vi "test-trapezoid-profile-timing-before-negative-goal.vi"() -> ()   [LabVIEW 2019]
uses:
  <vilib>/Rock Robotics/WPI/ThirdParty/JAS_Junk/TrajLib/TRAPEZOID_PROFILE_STATE.ctl
  <vilib>/Rock Robotics/WPI/ThirdParty/JAS_Junk/TrajLib/TRAPEZOID_PROFILE.ctl
  <vilib>/Rock Robotics/WPI/ThirdParty/JAS_Junk/TrajLib/TRAPEZOID_PROFILE_CONSTRAINT.ctl
  <vilib>/Rock Robotics/WPI/ThirdParty/JAS_Junk/TrajLib/TrapProfile_Direct.vi
  <vilib>/Rock Robotics/WPI/ThirdParty/JAS_Junk/TrajLib/TrapProfile_ShouldFlipAcceleration.vi
  <vilib>/Rock Robotics/WPI/ThirdParty/JAS_Junk/TrajLib/Trajectory_Library.lvlib
panel:
  out "ActualTime":dbl=-1.0
  out "PredictedTImeLeft":dbl
  out "TimeLeftGoal":dbl
  out "TimeLeftPos":dbl
  out "ReachedGoal":bool
  out "TotalTime":dbl
  out "TRAPEZOID_PROFILE":T1 {"Goal"."Velocity" format="%16_6e"; "Goal"."Position" format="%16_6e"; "Initial"."Velocity" format="%16_6e"; "Initial"."Position" format="%16_6e"; "Constraints"."MaxAcceleration" format="%16_6e"; "Constraints"."MaxVelocity" format="%16_6e"; "EndDecel" format="%16_6e"; "EndFullSpeed" format="%16_6e"; "EndAccel" format="%16_6e"}
  out "State":T3 {"Velocity" format="%16_6e"; "Position" format="%16_6e"}
  out "Waveform Chart":T4(graph)
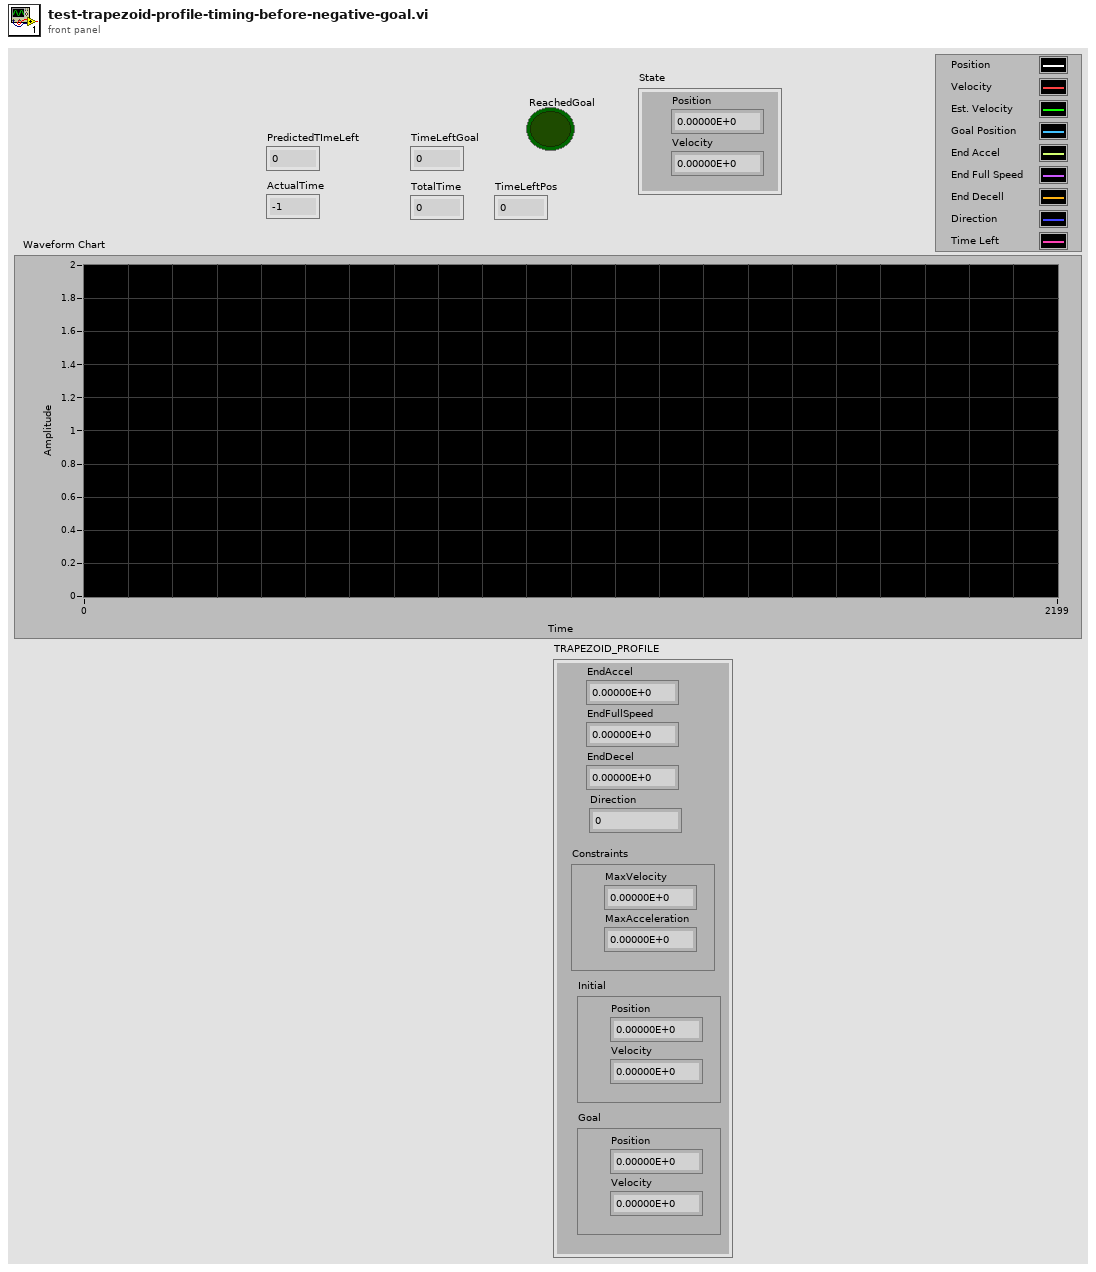
[diagram p1: front panel]
types:
  T1 = typedef "Trajectory_Library.lvlib/TRAPEZOID_PROFILE.ctl" = cluster{"EndAccel":dbl, "EndFullSpeed":dbl, "EndDecel":dbl, "Direction":i32, "Constraints":T2, "Initial":T3, "Goal":T3}
  T2 = typedef "Trajectory_Library.lvlib/TRAPEZOID_PROFILE_CONSTRAINT.ctl" = cluster{"MaxVelocity":dbl, "MaxAcceleration":dbl}
  T3 = typedef "Trajectory_Library.lvlib/TRAPEZOID_PROFILE_STATE.ctl" = cluster{"Position":dbl, "Velocity":dbl}
  T4 = cluster{"Position":dbl, "Velocity":dbl, dbl, "Position":dbl, "EndAccel":dbl, "EndFullSpeed":dbl, "EndDecel":dbl, "Direction":i32, "Position":dbl}
  T5 = cluster{"Position":dbl, "Velocity":dbl, dbl, "Position":dbl, "EndAccel":dbl, "EndFullSpeed":dbl, "EndDecel":dbl, "Direction":i32, "TimeLeft":dbl}
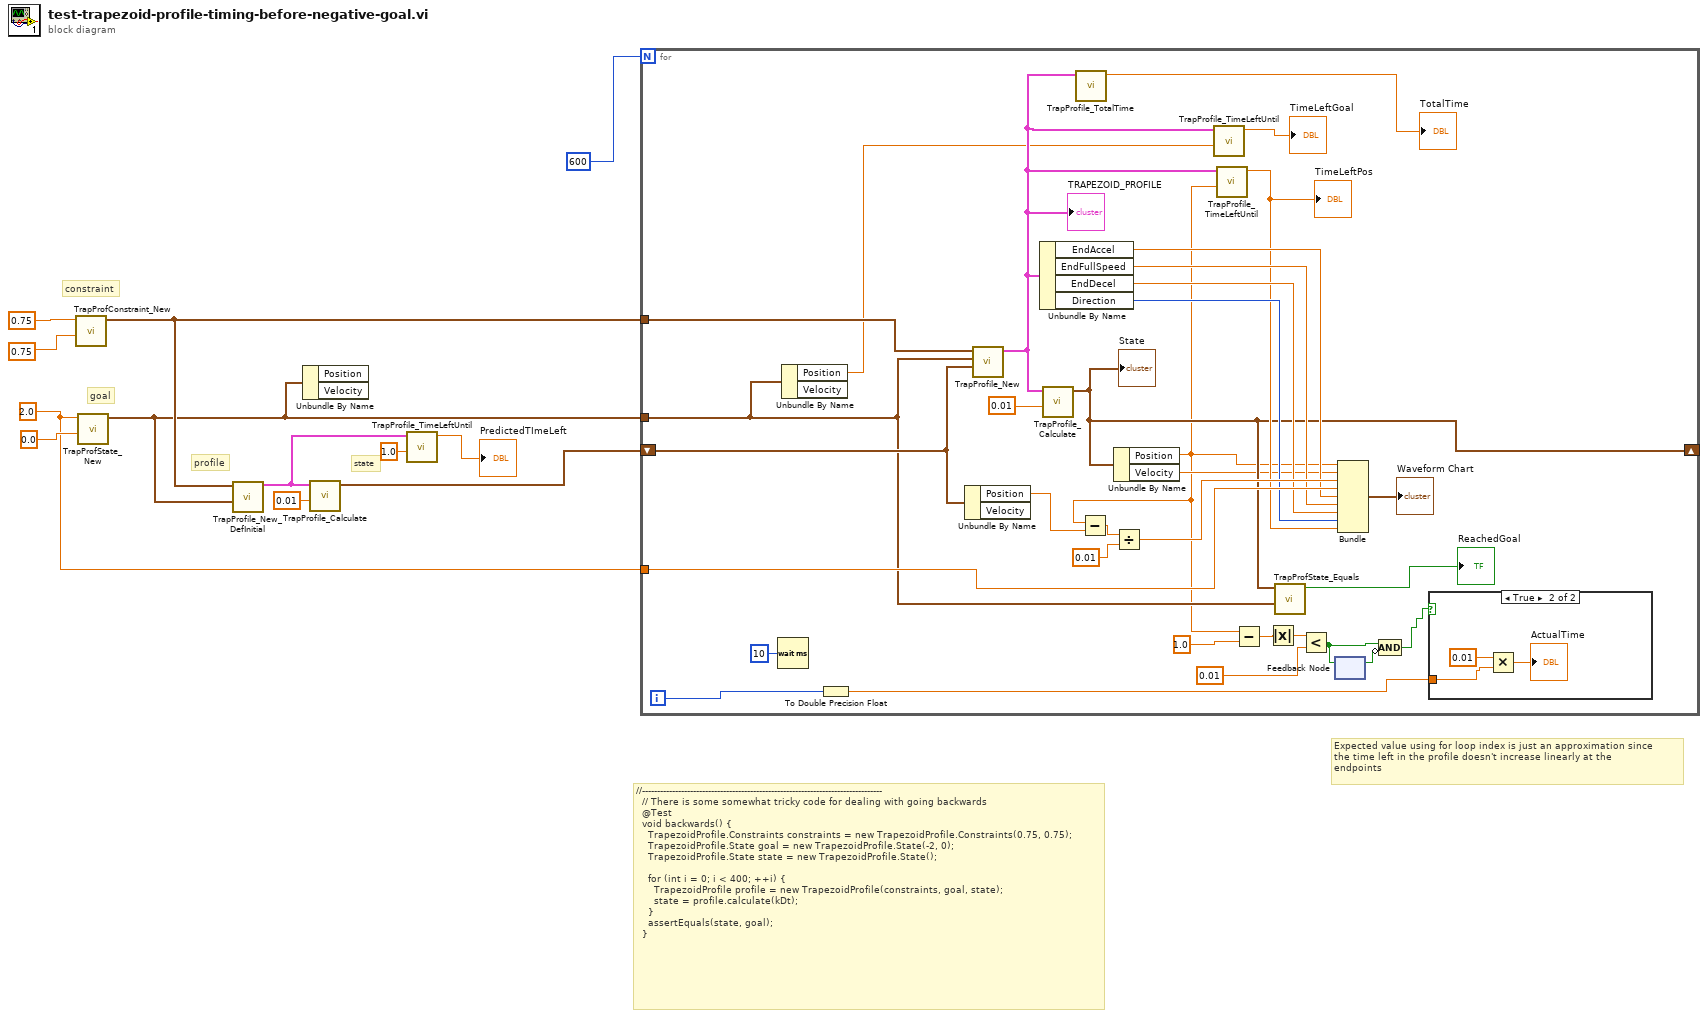
[diagram p0: block diagram]
diagram:
  w8 = 2.0 ("Position")
  # "Expected value using for loop index is just an approximation since\nthe time left in the profile doesn't increase linearly at the\nendpoints"
  # "profile"
  # "state"
  # "//--------------------------------------------------------------------------------\n  // There is some somewhat tricky code for dealing with going backwards\n  @Test\n  void backwards() {\n    TrapezoidProfile.Constraints constraints = new TrapezoidProfile.Constraints(0.75, 0.75);\n    TrapezoidProfile.State goal = new TrapezoidProfile.State(-2, 0);\n    TrapezoidProfile.State state = new TrapezoidProfile.State();\n\n    for (int i = 0; i < 400; ++i) {\n      TrapezoidProfile profile = new TrapezoidProfile(constraints, goal, state);\n      state = profile.calculate(kDt);\n    }\n    assertEquals(state, goal);\n  }"
  # "goal"
  # "constraint"
  n1 = call <vilib>:"TrapProfConstraint_New.vi"("Max Accel"=0.75, "Max Speed (M/S)"=0.75) -> ("TRAPEZOID_PROFILE_CONSTRAINT"=w7:T2)  [unwired: 9 in]
  n2 = call <vilib>:"TrapProfState_New.vi"("Velocity"=0.0, "Position"=w8) -> ("TRAPEZOID_PROFILE_STATE"=w4:T3)  [unwired: 9 in]
  n3 = call <vilib>:"TrapProfile_New_DefInitial.vi"("Goal"=w4, "Constraints"=w7) -> ("TRAPEZOID_PROFILE"=w3:T1)  [unwired: 9 in]
  n4 = Unbundle By Name(w4) -> ()  [unwired: 2 out]
  n5 = call <vilib>:"TrapProfile_Calculate.vi"("Time"=0.01, "TRAPEZOID_PROFILE"=w3) -> ("State"=w5:T3)  [unwired: 9 in]
  n6 = call <vilib>:"TrapProfile_TimeLeftUntil.vi"("TargetDistance"=1.0, "TRAPEZOID_PROFILE"=w3) -> ("TimeLeft"=→"PredictedTImeLeft":dbl)  [unwired: 9 in]
  n7 = for {
    N: 600 -> [_]
    shift-right: [w29] -> _
    shift-left: w5 -> [w42]
    tunnel: w4 -> [w26]
    tunnel: w8 -> [w38]
    tunnel: w7 -> [w32]
    i -> [w24]
    n8 = Wait (ms)(milliseconds to wait=u32 10) -> ()  [unwired: 1 out]
    n9 = Unbundle By Name(w26) -> ("Position"=w25:dbl)  [unwired: 1 out]
    n10 = To Double Precision Float(number=w24) -> (double precision float=w23:dbl)
    n11 = Unbundle By Name(w42) -> ("Position"=w33:dbl)  [unwired: 1 out]
    n12 = call <vilib>:"TrapProfile_New.vi"("Initial"=w42, "Goal"=w26, "Constraints"=w32) -> ("TRAPEZOID_PROFILE"=w28:T1)  [unwired: 8 in]
    "TRAPEZOID_PROFILE" <- w28
    n13 = Unbundle By Name(w28) -> ("EndAccel"=w37:dbl, "EndFullSpeed"=w36:dbl, "EndDecel"=w35:dbl, "Direction"=w34:i32)
    n14 = call <vilib>:"TrapProfile_Calculate.vi"("Time"=0.01, "TRAPEZOID_PROFILE"=w28) -> ("State"=w29:T3)  [unwired: 9 in]
    "State" <- w29
    n15 = call <vilib>:"TrapProfile_TotalTime.vi"("TRAPEZOID_PROFILE"=w28) -> ("TotalTime"=→"TotalTime":dbl)  [unwired: 10 in]
    n16 = Unbundle By Name(w29) -> ("Position"=w13:dbl, "Velocity"=w21:dbl)
    n17 = Subtract(x=w13, y=w33) -> (x-y=w41:dbl)
    n18 = Divide(x=w41, y=0.01) -> (x/y=w39:dbl)
    n19 = call <vilib>:"TrapProfile_TimeLeftUntil.vi"("TargetDistance"=w25, "TRAPEZOID_PROFILE"=w28) -> ("TimeLeft"=→"TimeLeftGoal":dbl)  [unwired: 9 in]
    n20 = call <vilib>:"TrapProfile_TimeLeftUntil.vi"("TargetDistance"=w13, "TRAPEZOID_PROFILE"=w28) -> ("TimeLeft"=w31:dbl)  [unwired: 9 in]
    "TimeLeftPos" <- w31
    n21 = Subtract(x=w13, y=1.0) -> (x-y=w19:dbl)
    n22 = Absolute Value(x=w19) -> (abs(x)=w18:dbl)
    n23 = call <vilib>:"TrapProfState_Equals.vi"("TRAPEZOID_PROFILE_STATE 2"=w26, "TRAPEZOID_PROFILE_STATE"=w29) -> ("Equal"=→"ReachedGoal":bool)  [unwired: 9 in]
    n24 = Less?(x=w18, y=0.01) -> (x < y?=w15:bool)
    n25 = feedback-in #1(w15) -> ()
    n26 = feedback #1() -> (w16:bool)  [unwired: 1 in]
    n27 = Bundle("Position"=w13, "Velocity"=w21, w39, "Position"=w38, "EndAccel"=w37, "EndFullSpeed"=w36, "EndDecel"=w35, "Direction"=w34, "TimeLeft"=w31) -> (→"Waveform Chart":T5)  [unwired: 1 in]
    n28 = Compound Arithmetic op=AND(w15, invert w16) -> (w14:bool)
    n29 = case shown="True" w14 {
      tunnel: w23 -> [_ w48]
      frame False {
      }
      frame True {
        n30 = Multiply(x=0.01, y=w48) -> (x*y=→"ActualTime":dbl)
      }
    }
  }
